vi "XML Script - Terminal.vi"(1 "location":T1, 2 "out":i32=-1, 4 "inName":string, 6 "name":string, 9 "prefix (name)":string, 10 "in":i32=-1) -> (5 "name (wire source)":string, 7 "XML Script Command - Control":string)   [LabVIEW 2017]
uses:
  <vilib>/_script/XML Scripting/Structure Location.ctl
  <vilib>/_script/XML Scripting/XML Script Tag.ctl
  <vilib>/_script/XML Scripting/XML Script Attribute.ctl
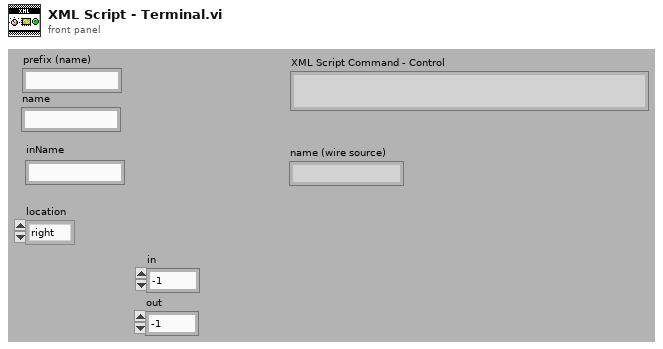
[diagram p1: front panel]
types:
  T1 = typedef "Structure Location.ctl" = enum16{"right", "left", "top", "bottom"}
  T2 = typedef "XML Script Attribute.ctl" = enum16{"name", "style", "path", "position", "in", "out", "width", "height", "index", "value", "default", "location", "offset", "typeindex", "size", "source", "destination", "indicator", "type", "controlname", "label", "conpaneidx", "mode", "description", "hasCondTerm", "linkIdentity", "caseselectortype", "concatInputs", "inName", "instantiationpath", "loopCondition", "IndexMode", "formulaInputs", "formulaOutputs", "msnFuncName", "msnIsDynamic", "msnIsODEUserFunction", "ignoreSearchDialog"}
  T3 = typedef "XML Script Tag.ctl" = enum16{"Script", "Function", "SubVI", "GrowableFunction", "Structure", "MultiframeStructure", "Frame", "Tunnel", "ShiftRegister", "Constant", "Control", "Terminal", "Wire", "StaticVIReference", "ControlTerminal", "CompoundArithmetic", "FlatSequence", "FlatSequenceFrame", "MathScriptCallByRef", "BuildArray", "GenericSubVI", "MathScriptNode"}
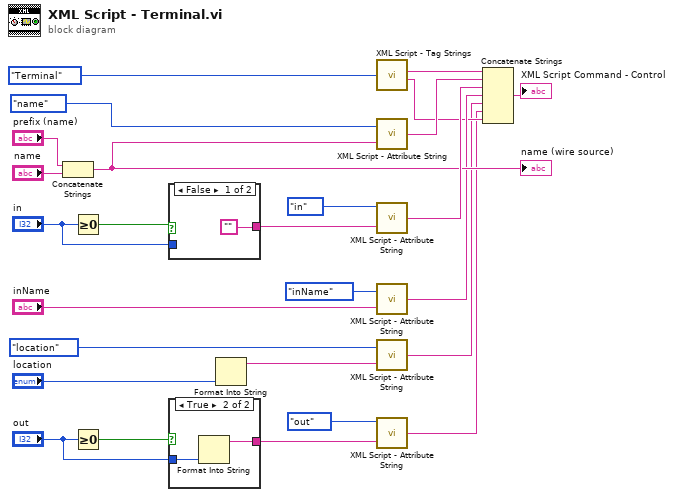
[diagram p0: block diagram]
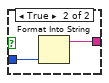
[diagram p2: hidden frame]
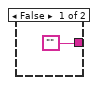
[diagram p3: hidden frame]
diagram:
  n1 = Concatenate Strings("prefix (name)", "name") -> (w13:string)
  "name (wire source)" <- w13
  n2 = Greater Or Equal To 0?(x="in") -> (x >= 0?=w9:bool)
  n3 = Greater Or Equal To 0?(x="out") -> (x >= 0?=w21:bool)
  n4 = case shown="False" w9 {
    tunnel: "in" -> [_ w29]
    tunnel: ["" w28] -> w17
    frame False {
    }
    frame True {
      n5 = Format Into String(w29) -> (resulting string=w28:string)  [unwired: 3 in, 1 out]
    }
  }
  n6 = case shown="True" w21 {
    tunnel: "out" -> [_ w32]
    tunnel: ["" w31] -> w18
    frame False {
    }
    frame True {
      n7 = Format Into String(w32) -> (resulting string=w31:string)  [unwired: 3 in, 1 out]
    }
  }
  n8 = Format Into String("location") -> (resulting string=w2:string)  [unwired: 3 in, 1 out]
  n9 = call <vilib>:"XML Script - Tag Strings.vi"("XML Script Tag"=XML_Script_Tag."Terminal") -> ("XML String - Begin Tag"=w24:string, "XML String - End Tag"=w6:string)  [unwired: 2 out]
  n10 = call <vilib>:"XML Script - Attribute String.vi"("Attribute String"=w13, "XML Script Attribute"=XML_Script_Attribute."name") -> ("XML Script - Attribute String"=w22:string)
  n11 = call <vilib>:"XML Script - Attribute String.vi"("Attribute String"=w17, "XML Script Attribute"=XML_Script_Attribute."in") -> ("XML Script - Attribute String"=w14:string)
  n12 = call <vilib>:"XML Script - Attribute String.vi"("Attribute String"="inName", "XML Script Attribute"=XML_Script_Attribute."inName") -> ("XML Script - Attribute String"=w10:string)
  n13 = call <vilib>:"XML Script - Attribute String.vi"("Attribute String"=w2, "XML Script Attribute"=XML_Script_Attribute."location") -> ("XML Script - Attribute String"=w1:string)
  n14 = call <vilib>:"XML Script - Attribute String.vi"("Attribute String"=w18, "XML Script Attribute"=XML_Script_Attribute."out") -> ("XML Script - Attribute String"=w5:string)
  n15 = Concatenate Strings(w24, w22, w14, w10, w1, w5, w6) -> (→"XML Script Command - Control":string)
